vi "create_new_configuration_item.vi"(8 "error in (no error)":errorcluster) -> (0 "error out":errorcluster, 1 "new-component config name out":string, 2 "component path out":path, 4 "canceled?":bool)   [LabVIEW 2010]
panel:
  in  "button: cancel":bool
  in  "button: ok":bool
  in  "component path":path
  in  "new-component config name":string caption="configuration name"
  # "Create configuration for component that is not yet listed"
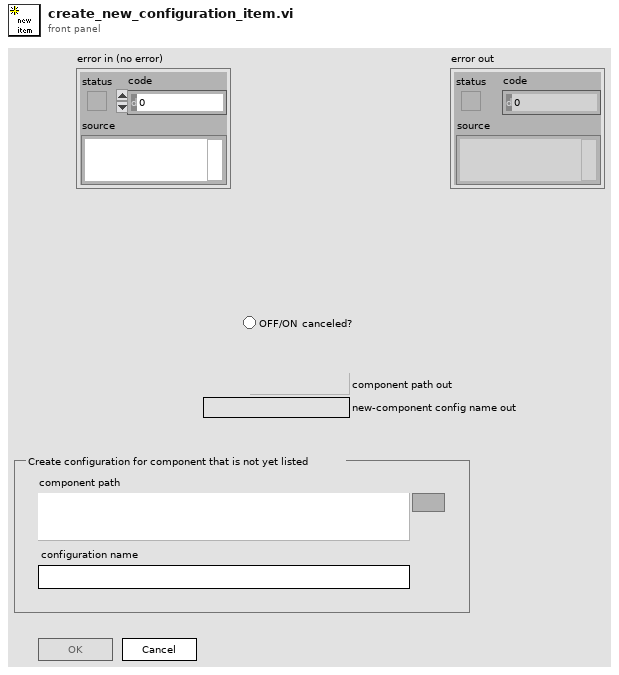
[diagram p1: front panel]
types:
  T1 = enum8{"Enabled", "Disabled", "Disabled and Grayed Out"}
  T2 = typedef "component_path_clusters.ctl" = cluster{"components directory":path, "component type directory":path, "specific component directory":path, "component class path":path}
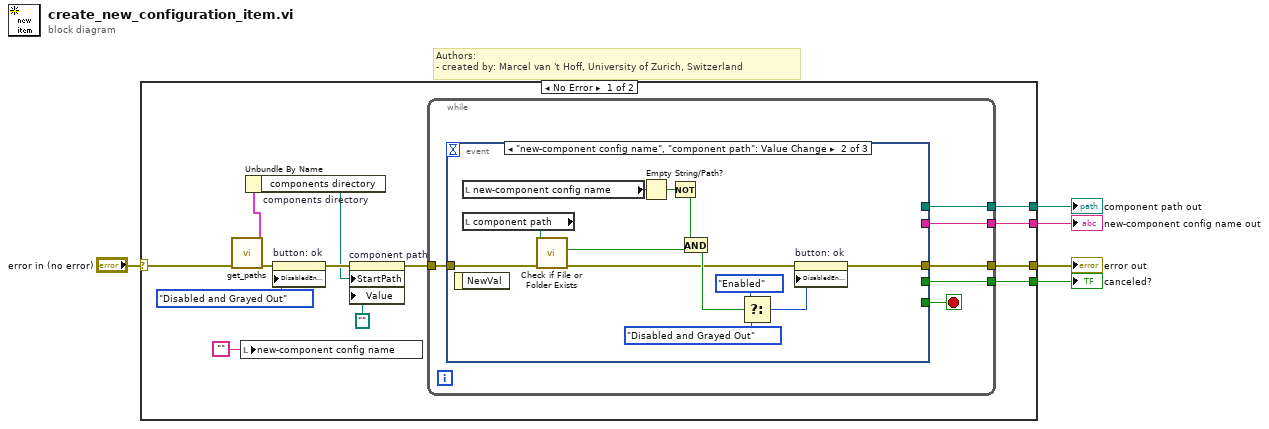
[diagram p0: block diagram]
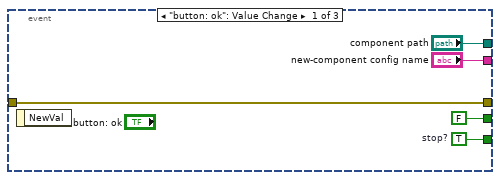
[diagram p2: hidden frame]
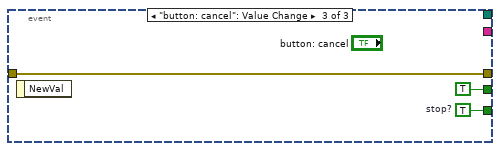
[diagram p3: hidden frame]
diagram:
  # "Authors: \n- created by: Marcel van 't Hoff, University of Zurich, Switzerland"
  n1 = case shown="No Error" "error in (no error)" {
    selector: "error in (no error)" -> [w12 w45]
    tunnel: [w18 w45] -> w5
    tunnel: [w17 _] -> w4
    tunnel: [w16 _] -> w3
    tunnel: [w15 _] -> w2
    frame No Error {
      n2 = call "get_paths.vi"("error in (no error)"=w12) -> ("error out"=w11:errorcluster, "component paths"=w13:T2)  [unwired: 7 in, 2 out]
      n3 = local write "new-component config name"("") -> ()
      n4 = Unbundle By Name "components directory"(w13) -> ("components directory"=w8:path)
      n5 = property on="button: ok" class="Bool"(error in=w11, "DisabledEnum"=T1."Disabled and Grayed Out" ("Disabled")) -> (error out=w10:errorcluster)  [unwired: 1 in, 1 out]
      n6 = property on="component path" class="Path"(error in=w10, "StartPath"=w8, "Value"=path "") -> (error out=w9:errorcluster)  [unwired: 1 in, 1 out]
      n7 = while {
        tunnel: [w24] -> w18
        tunnel: w9 -> [w23]
        tunnel: [w22] -> w17
        tunnel: [w21] -> w16
        tunnel: [w20] -> w15
        stop <- w19 stop-if-true
        n8 = event shown="[1] \"new-component config name\", \"component path\": Value Change" {
          selector: _ -> [_ _ _]
          dyn-events: _ -> [_ _ _]
          timeout: _ -> [_ _ _]
          tunnel: [w29 w31 w44] -> w24
          tunnel: w23 -> [w29 w40 w44]
          tunnel: [FALSE _ TRUE] -> w22
          tunnel: ["component path" _ _] -> w21
          tunnel: ["new-component config name" _ _] -> w20
          tunnel: [w25 _ w42] -> w19
          event "button: ok": Value Change {
            w25 = TRUE  # stop?
            n9 = event-data() -> ()  [unwired: 1 in, 1 out]
          }
          event "new-component config name", "component path": Value Change {
            n10 = event-data() -> ()  [unwired: 1 in, 1 out]
            n11 = local read "new-component config name"() -> (w36:string)
            n12 = local read "component path"() -> (w41:path)
            n13 = call <vilib>:"Check if File or Folder Exists.vi"("error in (no error)"=w40, "path"=w41) -> ("error out"=w32:errorcluster, "file or folder exists?"=w35:bool)  [unwired: 8 out]
            n14 = Empty String/Path?(string/path=w36) -> (empty?=w39:bool)
            n15 = Not(x=w39) -> (.not. x?=w34:bool)
            n16 = And(x=w34, y=w35) -> (x .and. y?=w38:bool)
            n17 = Select(t=T1."Enabled" ("Disabled"), s=w38, f=T1."Disabled and Grayed Out") -> (s? t:f=w30:T1)
            n18 = property on="button: ok" class="Bool"(error in=w32, "DisabledEnum"=w30) -> (error out=w31:errorcluster)  [unwired: 1 in, 1 out]
          }
          event "button: cancel": Value Change {
            w42 = TRUE  # stop?
            n19 = event-data() -> ()  [unwired: 1 in, 1 out]
          }
        }
      }
    }
    frame Error {
    }
  }
  "error out" <- w5
  "canceled?" <- w4
  "component path out" <- w3
  "new-component config name out" <- w2
